vi "Move Axis to Position.vi"(7 "error in (no error)":errorcluster, 8 "Position [internal units]":dbl format="%#_8f", 9 "Axis":T1, 10 "VISA in":refnum<visa-resource-name>) -> (0 "error out":errorcluster, 3 "VISA out":refnum<visa-resource-name>)   [LabVIEW 2018, in "ASI TG-1000.lvlib"]
doc: "Tells the ASI controller to move the (single) specified axis to the corresponding specified position; the equivalent of using the MOVE command. Note that it performs no checking to see if the move completes successfully."
uses:
  ASI TG-1000.lvlib
  Utility/Axis Name.ctl
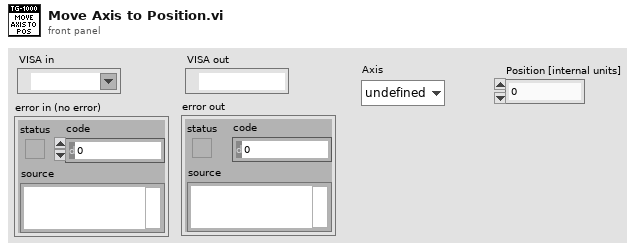
[diagram p1: front panel]
types:
  T1 = typedef "ASI TG-1000.lvlib/Axis Name.ctl" = enum8{"undefined", "A", "B", "C", "D", "E", "F", "G", "H", "I", "J", "K", "L", "M", "N", "O", "P", "Q", "R", "S", "T", "U", "V", "W", "X", "Y", "Z"}
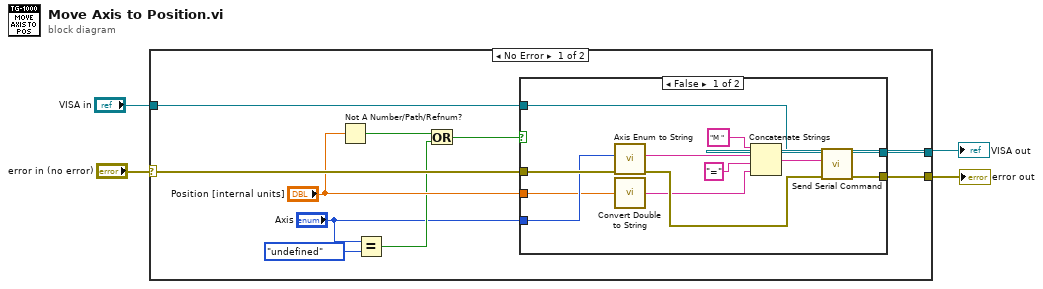
[diagram p0: block diagram]
diagram:
  n1 = case shown="No Error" "error in (no error)" {
    selector: "error in (no error)" -> [w13 w30]
    tunnel: "VISA in" -> [w14 w29]
    tunnel: [w12 w30] -> w2
    tunnel: [w11 w29] -> w1
    frame No Error {
      n2 = Not A Number/Path/Refnum?(number/path/refnum="Position [internal units]") -> (NaN/Path/Refnum?=w8:bool)
      n3 = Equal?(x="Axis", y=Axis_Name."undefined") -> (x = y?=w7:bool)
      n4 = Or(x=w8, y=w7) -> (x .or. y?=w6:bool)
      n5 = case shown="False" w6 {
        tunnel: "Position [internal units]" -> [w16 _]
        tunnel: w14 -> [w21 w27]
        tunnel: w13 -> [w20 w28]
        tunnel: [w19 w28] -> w12
        tunnel: [w18 w27] -> w11
        tunnel: "Axis" -> [w17 _]
        frame False {
          n6 = call "Axis Enum to String.vi"("error in (no error)"=w20, "Axis Enum In"=w17) -> ("error out"=w22:errorcluster, "Axis String Out"=w23:string)  [unwired: 8 in]
          n7 = call "Convert Double to String.vi"("Value"=w16) -> ("String"=w15:string)
          n8 = Concatenate Strings("M " ("Command"), w23, "=" ("string"), w15) -> (w25:string)
          n9 = call "Send Serial Command.vi"("error in (no error)"=w22, "Command"=w25, "VISA in"=w21) -> ("error out"=w19:errorcluster, "VISA out"=w18:refnum<visa-resource-name>)  [unwired: 6 in, 1 out]
        }
        frame True {
        }
      }
    }
    frame Error {
    }
  }
  "VISA out" <- w1
  "error out" <- w2
